vi "Do.vi"(8 "error in (no error)":errorcluster, 10 "Actor in":refnum<class "Actor.lvclass">, 11 "Save to TDMS Msg":refnum<class "Save to TDMS Msg.lvclass">) -> (0 "error out":errorcluster, 2 "Actor out":refnum<class "Actor.lvclass">)   [LabVIEW 2015, in "KIT-QA.lvlib" / "Save to TDMS Msg.lvclass"]
doc: "This VI delivers the message to the actor by calling the appropriate method(s) on the actor."
uses:
  Save to TDMS Msg.lvclass
  <vilib>/ActorFramework/Actor/Actor.lvclass
  KIT-QA/KIT-QA.lvclass
  Save to TDMS Msg.lvclass/Save to TDMS Msg.ctl
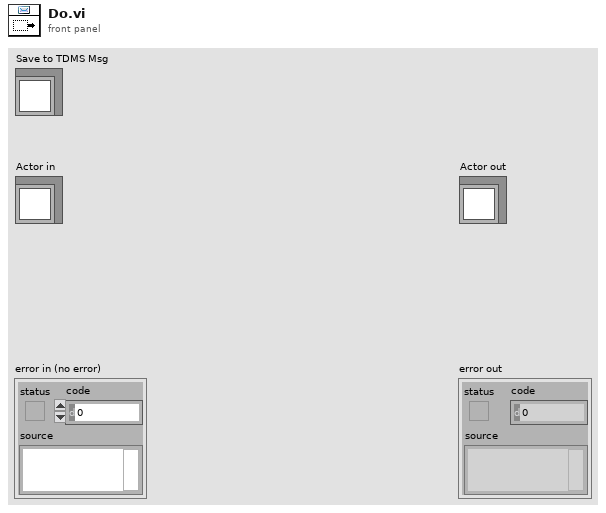
[diagram p1: front panel]
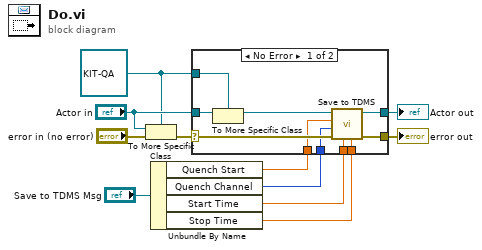
[diagram p0: block diagram]
diagram:
  w6 = refnum<class "KIT-QA.lvclass"> refnum ("Actor in")
  n1 = To More Specific Class(target class=w6, reference="Actor in", error in="error in (no error)") -> (error out=w10:errorcluster)  [unwired: 1 out]
  n2 = Unbundle By Name("Save to TDMS Msg") -> ("Quench Start"=w4:dbl[unit], "Quench Channel"=w3:i32, "Start Time"=w2:dbl[unit], "Stop Time"=w1:dbl[unit])
  n3 = case shown="No Error" w10 {
    selector: w10 -> [w19 w23]
    tunnel: [w21 w23] -> w9
    tunnel: [w20 w22] -> w8
    tunnel: "Actor in" -> [w18 w22]
    tunnel: w6 -> [w17 _]
    tunnel: w4 -> [w15 _]
    tunnel: w3 -> [w14 _]
    tunnel: w2 -> [w13 _]
    tunnel: w1 -> [w12 _]
    frame No Error {
      n4 = To More Specific Class(target class=w17, reference=w18) -> (specific class reference=w16:refnum<class "KIT-QA.lvclass">)  [unwired: 1 in, 1 out]
      n5 = call "Save to TDMS.vi"("Stop Time"=w12, "Start Time"=w13, "Error In"=w19, "Quench Channel"=w14, "Quench Start"=w15, "KIT-QA in"=w16) -> ("Error Out"=w21:errorcluster, "KIT-QA out"=w20:refnum<class "KIT-QA.lvclass">)  [unwired: 4 in]
    }
    frame Error {
    }
  }
  "error out" <- w9
  "Actor out" <- w8
